vi "Trigger_SWEep.vi"(8 "Error":errorcluster caption="错误输入（无错误）", 10 "Sweep":string(combo), 11 "VISA resource name":refnum<visa-resource-name>) -> (0 "Error out":errorcluster, 2 "Sweep out":string(combo), 3 "VISA resource name out":refnum<visa-resource-name>)   [LabVIEW 2020]
doc: "触发模式"
panel:
  out "读取缓冲区":string
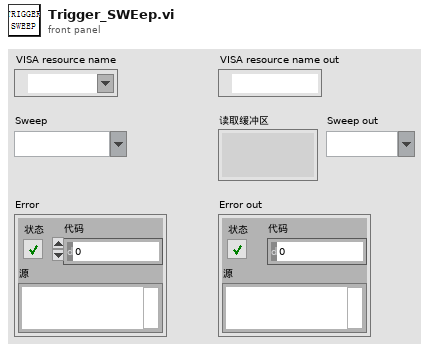
[diagram p1: front panel]
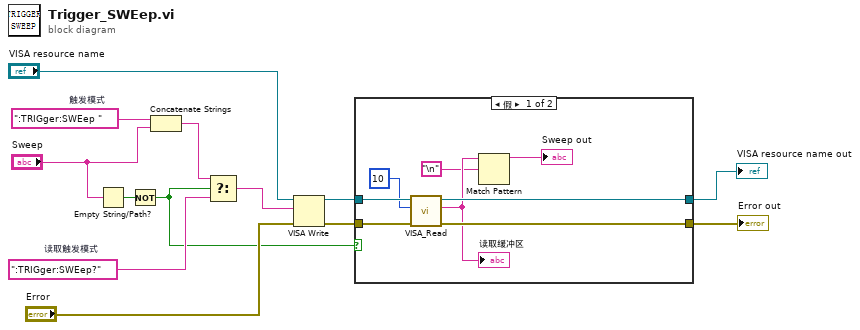
[diagram p0: block diagram]
diagram:
  w6 = ":TRIGger:SWEep?"  # 读取触发模式
  w12 = ":TRIGger:SWEep "  # 触发模式
  n1 = Empty String/Path?(string/path="Sweep") -> (empty?=w4:bool)
  n2 = Not(x=w4) -> (.not. x?=w3:bool)
  n3 = Concatenate Strings(w12, "Sweep") -> (w11:string)
  n4 = Select(t=w11, s=w3, f=w6) -> (s? t:f=w10:string)
  n5 = VISA Write(VISA resource name="VISA resource name", write buffer=w10, error in (no error)="Error") -> (VISA resource name out=w7:refnum<visa-resource-name>, error out=w9:errorcluster)  [unwired: 1 out]
  n6 = case shown="假" w3 {
    tunnel: w7 -> [w21 w23]
    tunnel: w9 -> [w20 w22]
    tunnel: [w18 w22] -> w8
    tunnel: [w19 w23] -> w1
    frame False {
      n7 = call "VISA_Read.vi"("Error"=w20, "字节总数"=u32 10, "VISA resource name"=w21) -> ("Error out"=w18:errorcluster, "读取缓冲区"=w17:string, "VISA resource name out"=w19:refnum<visa-resource-name>)  [unwired: 6 in]
      "读取缓冲区" <- w17
      n8 = Match Pattern(string=w17, regular expression="\n") -> (before substring=→"Sweep out":string)  [unwired: 1 in, 3 out]
    }
    frame True {
    }
  }
  "VISA resource name out" <- w1
  "Error out" <- w8
